vi "Monitor inquiry.vi"(0 "VISA resource name":refnum<visa-resource-name>, 1 "Channel  (1: CH1)":u16(ring)=1 items=["CH1"=1, "CH2"=2, "CH3"=3, "CH4"=4], 11 "error in (no error)":errorcluster) -> (3 "Stop Way":string, 4 "VISA resource name out":refnum<visa-resource-name>, 6 "Voltege":dbl, 8 "Current":dbl, 10 "Power":dbl, 12 "Voltqge Condition":string, 13 "Current Condition":string, 14 "Power Condition":string, 15 "error out":errorcluster)   [LabVIEW 2020, in "GPP.lvlib"]
uses:
  GPP.lvlib
  Function/VISA_COMMON.ctl
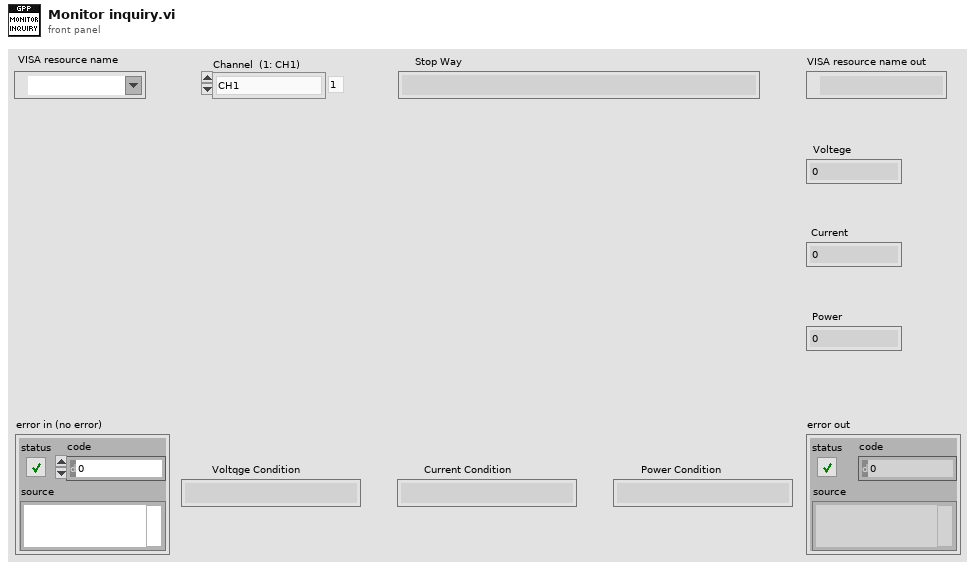
[diagram p1: front panel]
types:
  T1 = typedef "GPP.lvlib/VISA_COMMON.ctl" = enum16{"Initial", "Write CMD", "Read Result", "Read History", "Close"}
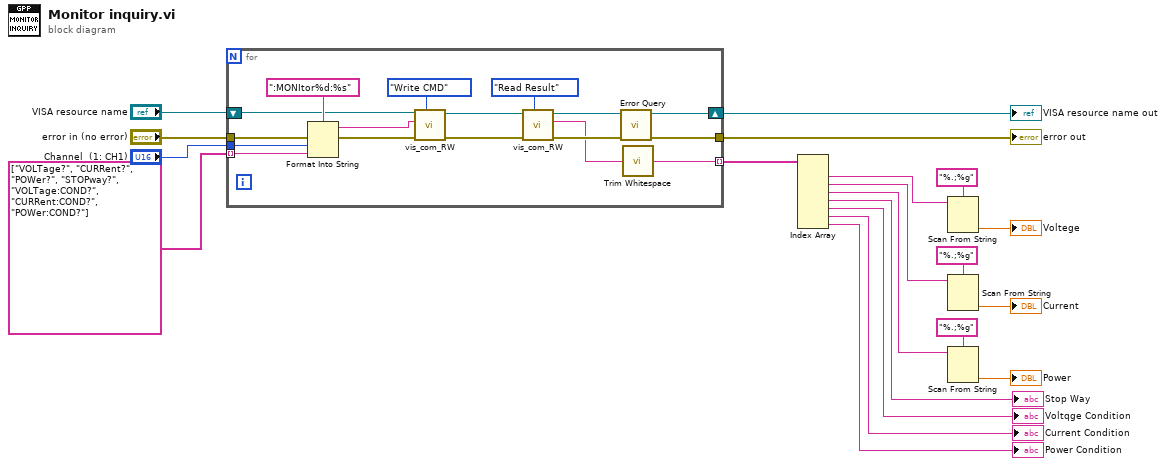
[diagram p0: block diagram]
diagram:
  n1 = for {
    tunnel: "error in (no error)" -> [w31]
    tunnel: "Channel  (1: CH1)" -> [w29]
    tunnel: string[] ["VOLTage?", "CURRent?", "POWer?", "STOPway?", "VOLTage:COND?", "CURRent:COND?", "POWer:COND?"] -> [w26] mode=indexing
    tunnel: [w27] -> w15
    tunnel: [w23] -> w17 mode=indexing
    shift-right: [w21] -> w14
    shift-left: "VISA resource name" -> [w25]
    n2 = Format Into String(format string=":MONItor%d:%s", error in=w31, w29, w26) -> (resulting string=w24:string, error out=w30:errorcluster)  [unwired: 1 in]
    n3 = call "vis_com_RW.vi"("Funciton"=VISA_COMMON."Write CMD", "error in (no error)"=w30, "CMD String"=w24, "VISA resource in"=w25) -> ("error out"=w35:errorcluster, "VISA resource out"=w34:refnum<visa-resource-name>)  [unwired: 5 in, 1 out]
    n4 = call "vis_com_RW.vi"("Funciton"=VISA_COMMON."Read Result", "error in (no error)"=w35, "VISA resource in"=w34) -> ("error out"=w32:errorcluster, "Result"=w22:string, "VISA resource out"=w33:refnum<visa-resource-name>)  [unwired: 6 in]
    n5 = call "Error Query.vi"("error in (no error)"=w32, "VISA resource name"=w33) -> ("error out"=w27:errorcluster, "VISA resource name out"=w21:refnum<visa-resource-name>)  [unwired: 6 in, 2 out]
    n6 = call <vilib>:"Trim Whitespace.vi"("string"=w22) -> ("trimmed string"=w23:string)  [unwired: 1 in]
  }
  "error out" <- w15
  "VISA resource name out" <- w14
  n7 = Index Array(array=w17) -> (element #1=w12:string, element #2=w9:string, element #3=w8:string, element #4=→"Stop Way":string, element #5=→"Voltqge Condition":string, element #6=→"Current Condition":string, element #7=→"Power Condition":string)  [unwired: 7 in]
  n8 = Scan From String(format string="%.;%g", input string=w12) -> (output 1=→"Voltege":dbl)  [unwired: 3 in, 3 out]
  n9 = Scan From String(format string="%.;%g", input string=w9) -> (output 1=→"Current":dbl)  [unwired: 3 in, 3 out]
  n10 = Scan From String(format string="%.;%g", input string=w8) -> (output 1=→"Power":dbl)  [unwired: 3 in, 3 out]
